vi "SENS_SEGM_ADD.vi"(0 "VISA IN":refnum<visa-resource-name>, 1 "Segment":i32, 5 "error in":errorcluster, 7 "Channel":i32) -> (14 "VISA Out":refnum<visa-resource-name>, 19 "error out":errorcluster)   [LabVIEW 2018, in "PNA-X.lvlib"]
doc: "SENSe<cnum>:SEGMent<snum>:ADD \n(Write-only) Adds a segment. \nParameters \n<cnum> Any existing channel number. If unspecified, value is set to 1 \n<snum> Segment number to add. If unspecified, value is set to 1. Segment numbers must \nbe sequential. If a new number is added where one currently exists, the existing \nsegment and those following are incremented by one. \nExamples Two Segments exist (1 and 2). The following command will add a new segment (1). The \nexisting (1 and 2) will become (2 and 3) respectively. \nSENS:SEGM1:ADD \nsense2:segment1:add \nQuery Syntax Not applicable. Use Sense:Segment:Count to determine the number of segments in a \ntrace. \nDefault Not Applicable"
uses:
  PNA-X.lvlib
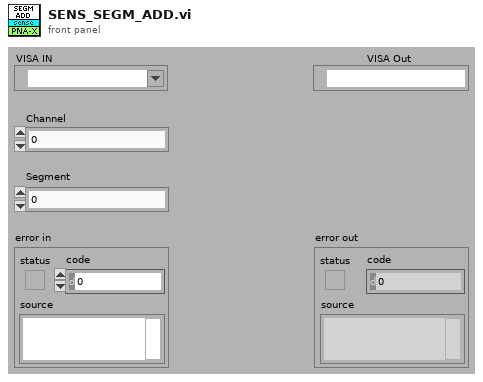
[diagram p1: front panel]
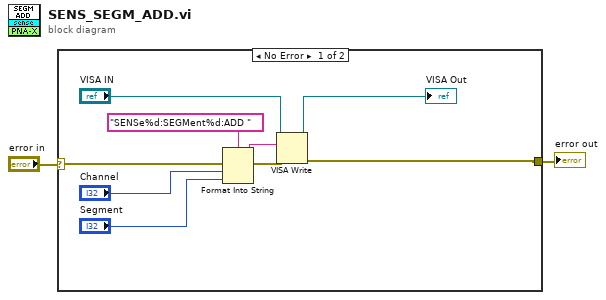
[diagram p0: block diagram]
diagram:
  n1 = case shown="No Error" "error in" {
    selector: "error in" -> [w11 w12]
    tunnel: [w6 w12] -> w1
    frame No Error {
      n2 = Format Into String(format string="SENSe%d:SEGMent%d:ADD " ("Cmdline"), error in=w11, "Channel", "Segment") -> (resulting string=w9:string, error out=w10:errorcluster)  [unwired: 1 in]
      n3 = VISA Write(VISA resource name="VISA IN", write buffer=w9, error in (no error)=w10) -> (VISA resource name out=→"VISA Out":refnum<visa-resource-name>, error out=w6:errorcluster)  [unwired: 1 out]
    }
    frame Error {
    }
  }
  "error out" <- w1
